vi "heinzCtrlGlobalsWrite.vi"(0 "w_postAccOffsetVoltControl":bool, 1 "postAccOffsetVoltControl":T1, 6 "w_postAccOffsetVoltState":bool, 7 "postAccOffsetVoltState":T1) -> ()   [LabVIEW 2014]
uses:
  Controls/heinzingerSelect.ctl
  <vilib>/rvi/Emulation/niFpgaSctlEmulationGetInTimedLoop.vi
  heinzingerControlGlobals.vi
  <vilib>/rvi/Emulation/niFpgaProcessEmulError.vi
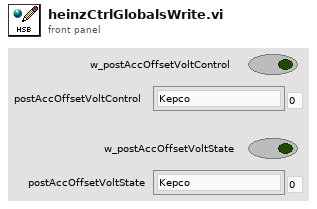
[diagram p1: front panel]
types:
  T1 = typedef "heinzingerSelect.ctl" = enum8{"Kepco", "Heinzinger0", "Heinzinger1", "Heinzinger2", "loading"}
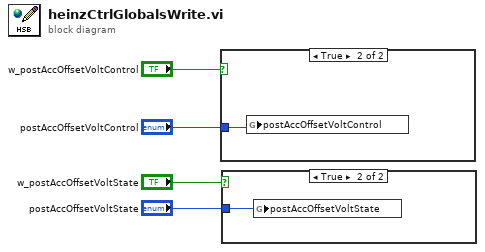
[diagram p0: block diagram]
diagram:
  n1 = case shown="True" "w_postAccOffsetVoltControl" {
    tunnel: "postAccOffsetVoltControl" -> [_ w5]
    frame False {
    }
    frame True {
      n2 = global write "heinzingerControlGlobals.vi" "postAccOffsetVoltControl"(w5) -> ()
    }
  }
  n3 = case shown="True" "w_postAccOffsetVoltState" {
    tunnel: "postAccOffsetVoltState" -> [_ w6]
    frame False {
    }
    frame True {
      n4 = global write "heinzingerControlGlobals.vi" "postAccOffsetVoltState"(w6) -> ()
    }
  }
